vi "tester2.vi"() -> ()   [LabVIEW 2009]
panel:
  out "s? t:f":dbl
  out "x >= y?":bool
  out "size(s)":i32
  out "Empty Array":T1(array[cluster])
  in  "stop":bool
  in  "Build Interval (ms)":dbl
  in  "Waveform Input":waveform(dbl)
  in  "Max Elapsed Build Time (ms)":dbl
  in  "Clear Trigger SP Latch":bool=TRUE
  in  "High Trigger SP (VDC)":dbl
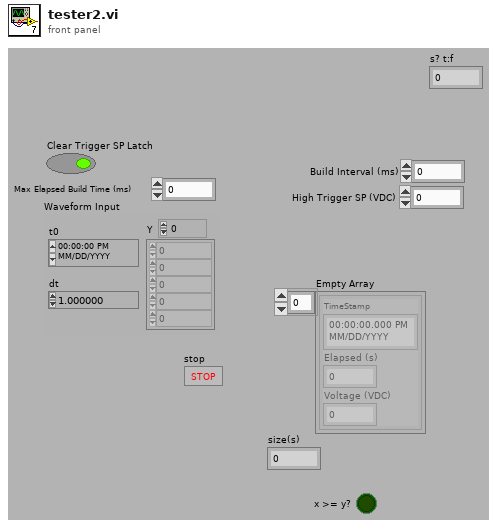
[diagram p1: front panel]
types:
  T1 = cluster{"TimeStamp":timestamp, "Elapsed (s)":dbl, "Voltage (VDC)":dbl}[]
  T2 = cluster{"TimeStamp":timestamp, "Elapsed (s)":dbl, "Voltage (VDC)":dbl}
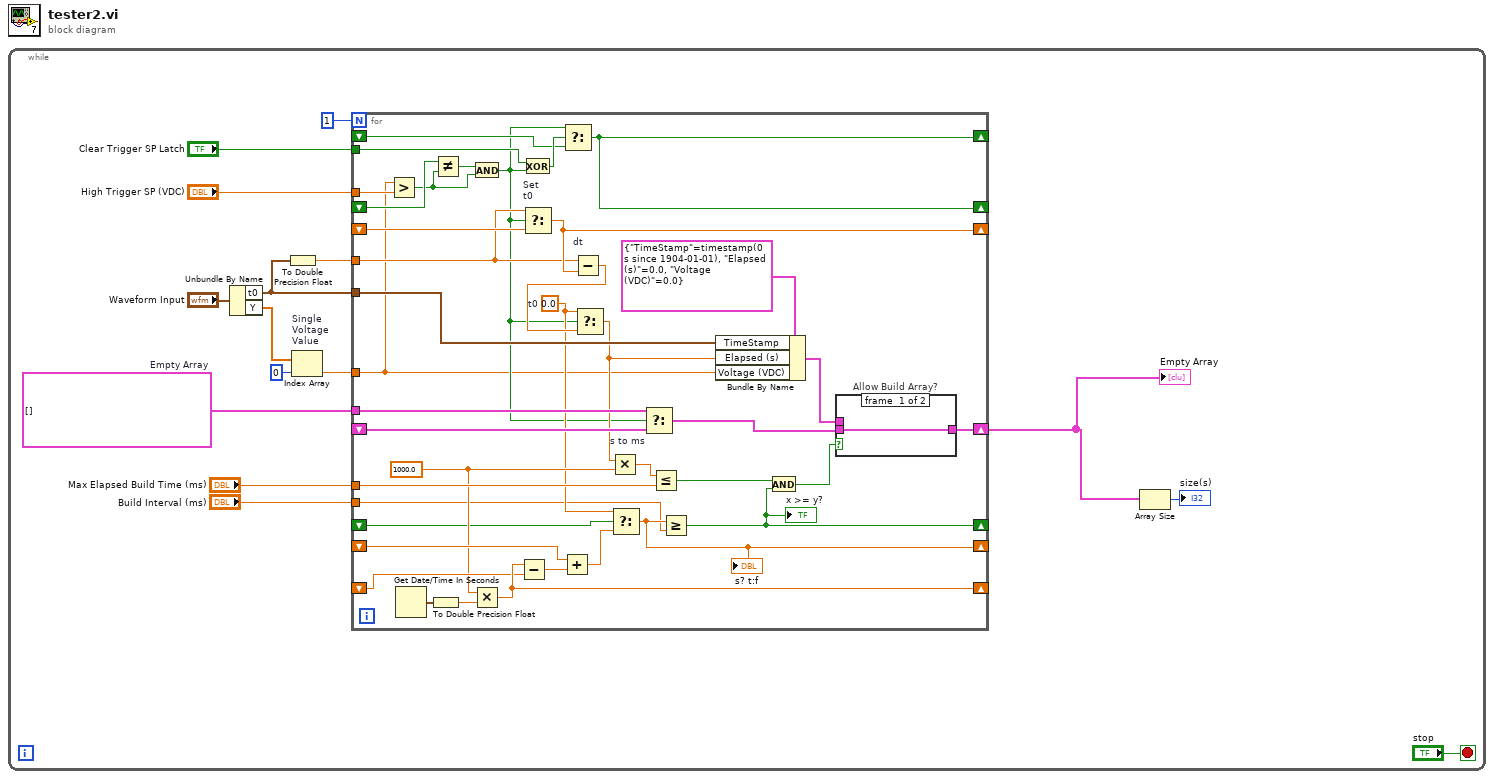
[diagram p0: block diagram]
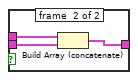
[diagram p2: hidden frame]
diagram:
  n1 = while {
    stop <- "stop" stop-if-true
    w9 = T1 []  # Empty Array
    n2 = Unbundle By Name("Waveform Input") -> ("t0"=w8:timestamp, "Y"=w11:dbl[])
    n3 = To Double Precision Float(number=w8) -> (double precision float=w7:dbl)
    n4 = Index Array "Single\nVoltage\nValue"(array=w11, index=0) -> (element=w10:dbl)
    n5 = for {
      N: 1 -> [_]
      tunnel: "High Trigger SP (VDC)" -> [w54]
      shift-right: [w46] -> _
      shift-left: _ -> [w52]
      shift-right: [w45] -> _
      shift-left: _ -> [w50]
      shift-right: [w46] -> _
      shift-left: _ -> [w48]
      tunnel: "Clear Trigger SP Latch" -> [w47]
      tunnel: w8 -> [w42]
      tunnel: w10 -> [w16]
      shift-right: [w40] -> w2
      shift-left: _ -> [w38]
      tunnel: w9 -> [w39]
      tunnel: w7 -> [w36]
      tunnel: "Max Elapsed Build Time (ms)" -> [w34]
      shift-right: [w29] -> _
      shift-left: _ -> [w28]
      shift-right: [w25] -> _
      shift-left: _ -> [w26]
      shift-right: [w18] -> _
      shift-left: _ -> [w20]
      tunnel: "Build Interval (ms)" -> [w21]
      w24 = 1000.0 ("y")
      w23 = 0.0  # t0
      n6 = Greater?(x=w16, y=w54) -> (0:w51:bool)
      n7 = Get Date/Time In Seconds() -> (seconds since 1Jan1904=w32:timestamp)
      n8 = To Double Precision Float(number=w32) -> (double precision float=w27:dbl)
      n9 = Not Equal?(x=w52, y=w51) -> (x != y?=w53:bool)
      n10 = And(x=w53, y=w51) -> (x .and. y?=w22:bool)
      n11 = Multiply(x=w24, y=w27) -> (x*y=w29:dbl)
      n12 = Subtract(x=w29, y=w28) -> (x-y=w31:dbl)
      n13 = Exclusive Or(1:w22, 2:w47) -> (0:w49:bool)
      n14 = Select "Set\nt0"(t=w36, s=w22, f=w50) -> (s? t:f=w45:dbl)
      n15 = Add(x=w26, y=w31) -> (x+y=w30:dbl)
      n16 = Select(t=w22, s=w49, f=w48) -> (s? t:f=w46:bool)
      n17 = Subtract "dt"(x=w36, y=w45) -> (x-y=w44:dbl)
      n18 = Select(t=w23, s=w22, f=w44) -> (s? t:f=w35:dbl)
      n19 = Multiply "s to ms"(x=w35, y=w24) -> (x*y=w33:dbl)
      n20 = Select(t=w23, s=w20, f=w30) -> (s? t:f=w25:dbl)
      "s? t:f" <- w25
      n21 = Select(t=w39, s=w22, f=w38) -> (s? t:f=w37:T1)
      n22 = Less Or Equal?(x=w33, y=w34) -> (x <= y?=w19:bool)
      n23 = Greater Or Equal?(x=w25, y=w21) -> (x >= y?=w18:bool)
      "x >= y?" <- w18
      n24 = Bundle By Name(cluster=T2 {"TimeStamp"=timestamp(0 s since 1904-01-01), "Elapsed (s)"=0.0, "Voltage (VDC)"=0.0}, "TimeStamp"=w42, "Elapsed (s)"=w35, "Voltage (VDC)"=w16) -> (w41:T2)
      n25 = And(x=w19, y=w18) -> (x .and. y?=w17:bool)
      n26 = case "Allow Build Array?" shown="True" w17 {
        tunnel: w41 -> [_ w58]
        tunnel: [w55 w57] -> w40
        tunnel: w37 -> [w55 w56]
        frame #0 {
        }
        frame #1 {
          n27 = Build Array (concatenate)(w58, w56) -> (w57:T1)
        }
      }
    }
    "Empty Array" <- w2
    n28 = Array Size(array=w2) -> (size(s)=→"size(s)":i32)
  }
